vi "Inspect Tell Self.vi"(4 "Priority":bool, 6 "Reply":bool, 8 "Error in":errorcluster, 9 "Msg in":refnum<class "Msg.lvclass">, 11 "TEMPLATE Actor in":refnum<class "TEMPLATE Actor.lvclass">) -> (0 "Error out":errorcluster, 1 "Msg out":refnum<class "Msg.lvclass">, 2 "Proceed":bool=TRUE, 3 "TEMPLATE Actor out":refnum<class "TEMPLATE Actor.lvclass">)   [LabVIEW 2020, in "_Template.lvlib" / "Templates.lvlib" / "TEMPLATE jettl Actor.lvlib" / "TEMPLATE Actor.lvlib" / "TEMPLATE Actor.lvclass"]
uses:
  TEMPLATE Actor.lvclass
  jettl/jettl/Msg/Msg.lvclass
  TEMPLATE Actor.lvclass/TEMPLATE Actor.ctl
  jettl/jettl/Actor/Actor.lvclass
panel:
  # "This front panel should not be manipulated."
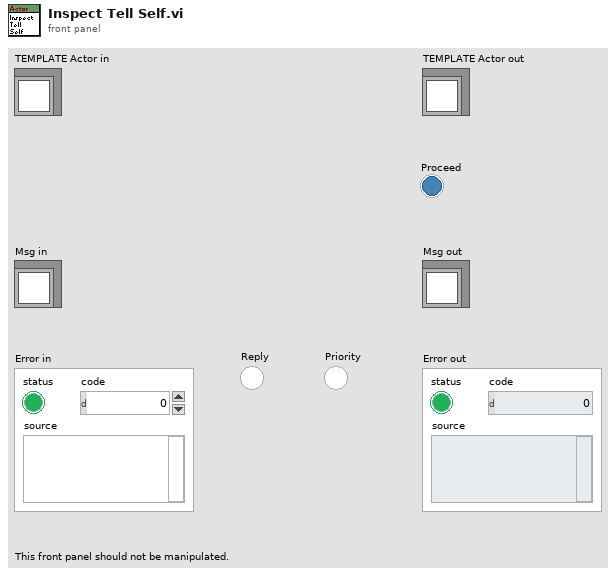
[diagram p1: front panel]
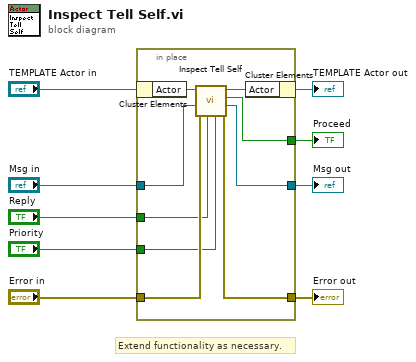
[diagram p0: block diagram]
diagram:
  # "Extend functionality as necessary."
  n1 = in-place {
    in-place-border: "Error in" -> [w15]
    in-place-border: "Msg in" -> [w16]
    in-place-border: "Reply" -> [w10]
    in-place-border: "Priority" -> [w11]
    in-place-border: [w14] -> w3
    in-place-border: [w13] -> w2
    in-place-border: [w12] -> w1
    n2 = in-place-cluster #1("TEMPLATE Actor in") -> ("Actor"=w18:refnum<class "Actor.lvclass">)
    n3 = call-dynamic "Inspect Tell Self.vi"("Priority"=w11, "Reply"=w10, "Error in"=w15, "Msg in"=w16, "Actor in"=w18) -> ("Error out"=w14:errorcluster, "Msg out"=w12:refnum<class "Msg.lvclass">, "Proceed"=w13:bool, "Actor out"=w17:refnum<class "Actor.lvclass">)  [unwired: 3 in]
    n4 = in-place-cluster #1("Actor"=w17) -> (→"TEMPLATE Actor out":refnum<class "TEMPLATE Actor.lvclass">)
  }
  "Proceed" <- w2
  "Error out" <- w3
  "Msg out" <- w1
